vi "Sequence.Load.vi"(8 "error in (no error)":errorcluster) -> (0 "error out":errorcluster, 2 "Sequence Data [ ]":T1[](array[typedef]), 3 "Sequence file path dup":path)   [LabVIEW 2019]
doc: "Prompts the user to select a sequence (CSV) file from disk, reads it, and then outputs Sequence Data [ ], which is an array of sequence steps."
uses:
  typedefs/step.data--Cluster.ctl
  typedefs/step.IO.data--Cluster.ctl
  typedefs/IOType--Enum.ctl
panel:
  out "cancelled?":bool
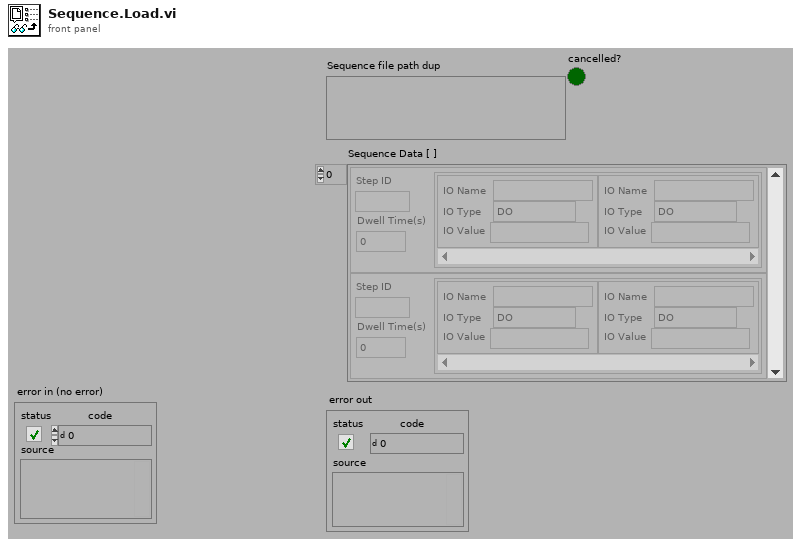
[diagram p1: front panel]
types:
  T1 = typedef "step.data--Cluster.ctl" = cluster{"Step ID":string, "Dwell Time(s)":dbl, "Recipe Step":T2[]}
  T2 = typedef "step.IO.data--Cluster.ctl" = cluster{"IO Name":string, "IO Type":T3, "IO Value":variant}
  T3 = typedef "IOType--Enum.ctl" = enum16{"<Undefined>", "DO", "DI", "AO", "AI"}
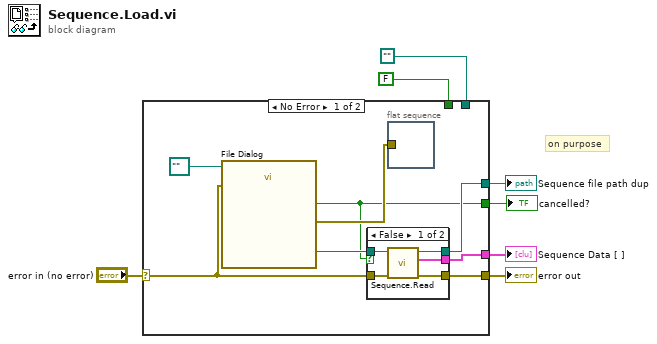
[diagram p0: block diagram]
diagram:
  # "on purpose"
  n1 = case shown="No Error" "error in (no error)" {
    selector: "error in (no error)" -> [w8 w25]
    tunnel: [w12 _] -> w7
    tunnel: [w11 w24] -> w6
    tunnel: [w10 w25] -> w5
    tunnel: [w9 w23] -> w4
    tunnel: path "" -> [_ w24]
    tunnel: FALSE -> [_ w23]
    frame No Error {
      n2 = call "File Dialog"("start path"=path "" ("Recipe file path"), "error in"=w8) -> ("selected path"=w13:path, "cancelled"=w9:bool, "error out"=w14:errorcluster)  [unwired: 10 in, 1 out]
      n3 = case shown="False" w9 {
        tunnel: w8 -> [w20 w22]
        tunnel: w13 -> [w19 w21]
        tunnel: [w18 _] -> w12
        tunnel: [w17 w21] -> w11
        tunnel: [w16 w22] -> w10
        frame False {
          n4 = call "Sequence.Read.vi"("error in (no error)"=w20, "Recipe file path"=w19) -> ("error out"=w16:errorcluster, "Recipe Data"=w18:T1[], "Recipe file path dup"=w17:path)  [unwired: 7 in]
        }
        frame True {
        }
      }
      n5 = flat-sequence {
        tunnel: w14 -> [_]
        frame #0 {
        }
      }
    }
    frame Error {
    }
  }
  "Sequence file path dup" <- w6
  "error out" <- w5
  "Sequence Data [ ]" <- w7
  "cancelled?" <- w4
